vi "Non Delay Scheduler Engine.vi"(8 "Number of  Jobs":i32=4, 9 "Number of Machines":i32=4, 10 "Processing Times":u16[][](array[numeric])=[[34, 15, 38, 95], [2, 89, 19, 7], [54, 70, 28, 34], [61, 9, 87, 29]], 11 "Schedule":u16[](array[numeric])=[12, 0, 7, 2, 6, 3, 13, 5, 1, 4, 14, 11, 10, 15, 8, 9]) -> (0 "Reordered Schedule":u16[](array[numeric]), 1 "Job Completion Times":u16[](array[numeric]), 2 "Completion Times":u16[][](array[numeric]), 3 "Start Times":u16[][](array[numeric]), 4 "Machine Completion Times":u16[](array[numeric]), 5 "Equal?":bool)   [LabVIEW 2013, in "Scheduler.lvclass"]
uses:
  Scheduler.lvclass
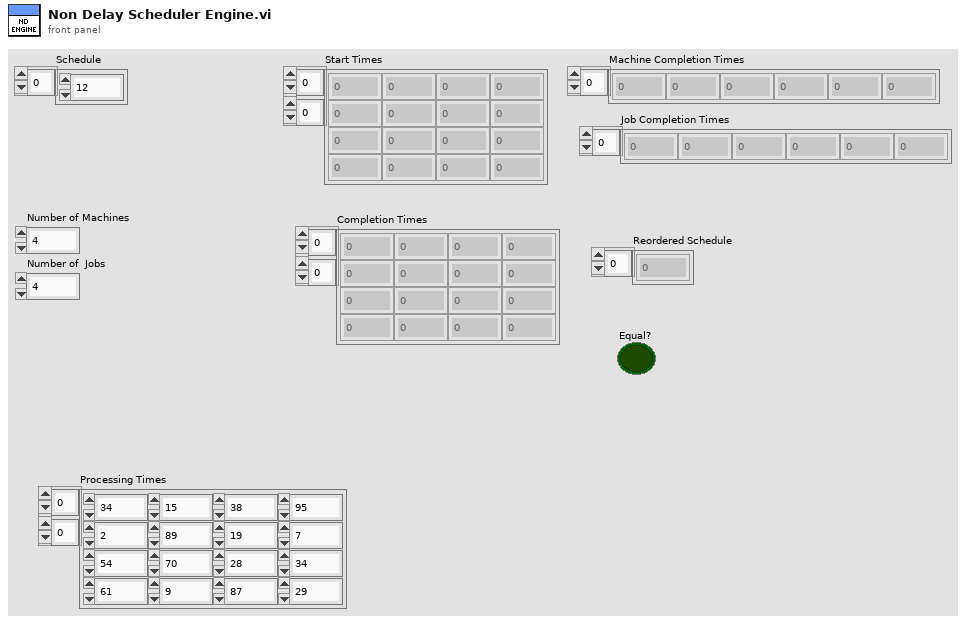
[diagram p1: front panel]
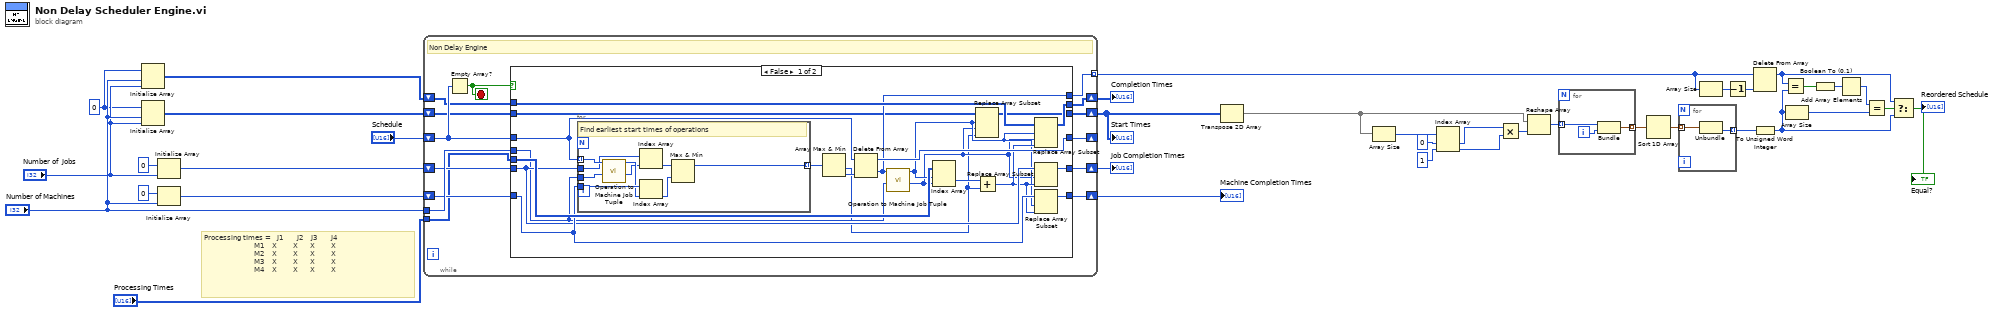
[diagram p0: block diagram]
diagram:
  w22 = u16 0 ("element")
  # "Processing tImes =   J1       J2    J3       J4   \n                         M1    X        X      X        X\n                         M2    X        X      X        X\n                         M3    X        X      X        X\n                         M4    X        X      X        X"
  n1 = Initialize Array(w22, "Number of Machines", "Number of  Jobs") -> (w32:u16[][])
  n2 = Initialize Array(w22, "Number of Machines", "Number of  Jobs") -> (w21:u16[][])
  n3 = Initialize Array(u16 0 ("element"), "Number of  Jobs") -> (w35:u16[])
  n4 = Initialize Array(u16 0 ("element"), "Number of Machines") -> (w34:u16[])
  n5 = while {
    shift-right: [w43] -> _
    shift-left: "Schedule" -> [w50]
    tunnel: "Number of Machines" -> [w49]
    shift-right: [w46] -> w30
    shift-left: w35 -> [w48]
    shift-right: [w45] -> w29
    shift-left: w34 -> [w47]
    shift-right: [w41] -> w31
    shift-left: w32 -> [w42]
    tunnel: "Processing Times" -> [w44]
    tunnel: [w40] -> w27 mode=indexing
    shift-right: [w38] -> w9
    shift-left: w21 -> [w39]
    stop <- w51 stop-if-true
    # "Non Delay Engine"
    n6 = Empty Array?(array=w50) -> (empty?=w51:bool)
    n7 = case shown="False" w51 {
      tunnel: w50 -> [w63 w83]
      tunnel: w49 -> [w58 _]
      tunnel: w48 -> [w69 w85]
      tunnel: w47 -> [w70 w84]
      tunnel: [w68 w85] -> w46
      tunnel: [w67 w84] -> w45
      tunnel: w44 -> [w71 _]
      tunnel: [w62 w83] -> w43
      tunnel: w42 -> [w66 w82]
      tunnel: [w65 w82] -> w41
      tunnel: [w57 _] -> w40
      tunnel: w39 -> [w56 w81]
      tunnel: [w52 w81] -> w38
      frame False {
        n8 = for {
          tunnel: w63 -> [w80] mode=indexing
          tunnel: w58 -> [w79]
          tunnel: w69 -> [w76]
          tunnel: w70 -> [w78]
          tunnel: [w72] -> w64 mode=indexing
          # "Find earliest start times of operations"
          n9 = call "Operation to Machine Job Tuple.vi"("Number of Machines"=w79, "Operation Number"=w80) -> ("Job No"=w75:i32, "Machine No"=w77:i32)  [unwired: 8 in]
          n10 = Index Array(array=w76, index=w75) -> (element=w74:u16)
          n11 = Index Array(array=w78, index=w77) -> (element=w73:u16)
          n12 = Max & Min(x=w74, y=w73) -> (max(x,y)=w72:u16)  [unwired: 1 out]
        }
        n13 = Array Max & Min(array=w64) -> (min value=w53:u16, min index (indices)=w59:i32)  [unwired: 2 out]
        n14 = Delete From Array(array=w63, index=w59) -> (deleted portion=w57:u16, array with subset deleted=w62:u16[])  [unwired: 1 in]
        n15 = call "Operation to Machine Job Tuple.vi"("Number of Machines"=w58, "Operation Number"=w57) -> ("Job No"=w54:i32, "Machine No"=w55:i32)  [unwired: 8 in]
        n16 = Index Array(array=w71, index (row)=w55, index (col)=w54) -> (element=w61:u16)
        n17 = Replace Array Subset(array=w56, new element=w53, index (row)=w55, index (col)=w54) -> (w52:u16[][])
        n18 = Add(x=w61, y=w53) -> (x+y=w60:u16)
        n19 = Replace Array Subset(array=w66, new element=w60, index (row)=w55, index (col)=w54) -> (w65:u16[][])
        n20 = Replace Array Subset(array=w69, new element=w60, index=w54) -> (w68:u16[])
        n21 = Replace Array Subset(array=w70, new element=w60, index=w55) -> (w67:u16[])
      }
      frame True {
      }
    }
  }
  "Completion Times" <- w31
  "Job Completion Times" <- w30
  "Machine Completion Times" <- w29
  "Start Times" <- w9
  n22 = Transpose 2D Array(2D array=w9) -> (transposed array=w15:u16[][])
  n23 = Array Size(array=w15) -> (size(s)=w20:i32[])
  n24 = Index Array(array=w20, index #1=0 ("index"), index #2=1 ("index")) -> (element #1=w17:i32, element #2=w16:i32)
  n25 = Multiply(x=w17, y=w16) -> (x*y=w14:i32)
  n26 = Reshape Array(w15, w14) -> (w13:u16[])
  n27 = for {
    tunnel: w13 -> [w88] mode=indexing
    tunnel: [w86] -> w12 mode=indexing
    i -> [w87]
    n28 = Bundle("element"=w88, w87) -> (w86:cluster{"element":u16, i32})  [unwired: 1 in]
  }
  n29 = Sort 1D Array(array=w12) -> (sorted array=w11:cluster{"element":u16, i32}[])
  n30 = for {
    tunnel: w11 -> [w90] mode=indexing
    tunnel: [w89] -> w10 mode=indexing
    n31 = Unbundle(w90) -> (w89:i32)  [unwired: 1 out]
  }
  n32 = Array Size(array=w27) -> (size(s)=w26:i32)
  n33 = Decrement(x=w26) -> (x-1=w25:i32)
  n34 = Delete From Array(array=w27, index=w25) -> (array with subset deleted=w3:u16[])  [unwired: 1 in, 1 out]
  n35 = To Unsigned Word Integer(number=w10) -> (unsigned 16bit integer=w2:u16[])
  n36 = Equal?(x=w3, y=w2) -> (x = y?=w8:bool[])
  n37 = Array Size(array=w2) -> (size(s)=w5:i32)
  n38 = Boolean To (0,1)(Boolean=w8) -> (0, 1=w7:i16[])
  n39 = Add Array Elements(numeric array=w7) -> (sum=w6:i16)
  n40 = Equal?(x=w6, y=w5) -> (x = y?=w4:bool)
  "Equal?" <- w4
  n41 = Select(t=w3, s=w4, f=w2) -> (s? t:f=→"Reordered Schedule":u16[])
